vi "Sort SRs per Week(SubVI).vi"(8 "error in (no error)":errorcluster, 10 "Weeks":u8[](array[numeric]), 11 "Data Value Reference in":refnum<data-value>) -> (0 "error out":errorcluster, 3 "DVR Weekly/Country Data":refnum<data-value>)   [LabVIEW 2017, in "DS_Lib.lvlib" / "SRReportParser.lvlib"]
uses:
  Modules/Private Controls/Report Data Cluster.ctl
  Modules/Private Controls/Data Raw.ctl
  TypeDefs/WeeklyData.ctl
  SRReportParser.lvlib
  Modules/Data Operations.lvlib
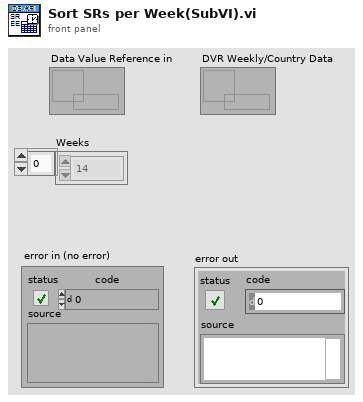
[diagram p1: front panel]
types:
  T1 = typedef "DS_Lib.lvlib/SRReportParser.lvlib/WeeklyData.ctl" = cluster{"Week":u8, "AE-Romania":T2[], "AE-Poland":T2[], "AE-Hungary":T2[], "AE-Czech and Slovakia":T2[]}
  T2 = typedef "Data Operations.lvlib/Data Raw.ctl" = cluster{"SR Number":string, "Status":string, "Summary":string, "AE Owner":string, "AE Group":string, "Contact":string, "SurveyData":cluster{"Resolution Time":dbl, "Total Satisfaction":dbl, "Response Time":dbl, "Courtesy":dbl, "Problem Solved":dbl, "Level of effort":dbl}, "Time Data":cluster{"Last Update Date":timestamp, "Creation Date":timestamp, "Creation week":u8, "Last Update Week":u8}}
  T3 = typedef "Data Operations.lvlib/Report Data Cluster.ctl" = cluster{"Headers":cluster{"Start Date":timestamp, "End Date":timestamp, "SR Status String":string[], "AE Owner String":string[]}, "Data":T2[]}
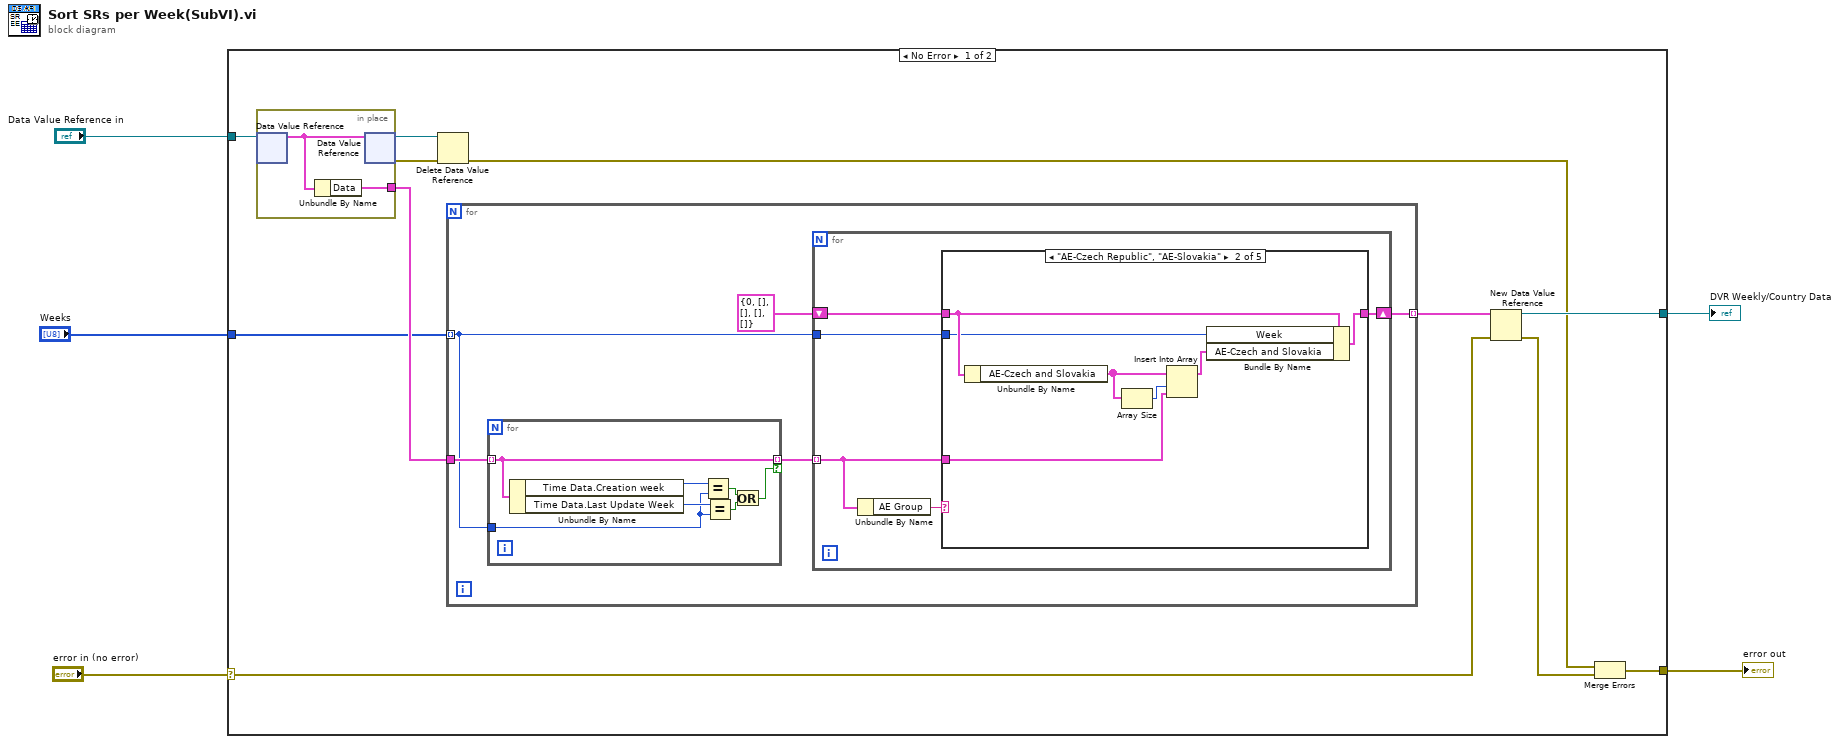
[diagram p0: block diagram]
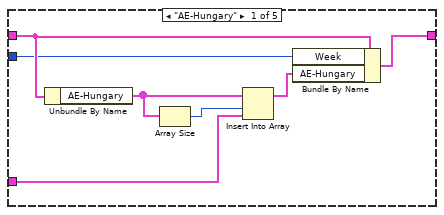
[diagram p2: hidden frame]
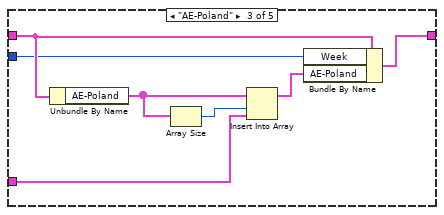
[diagram p3: hidden frame]
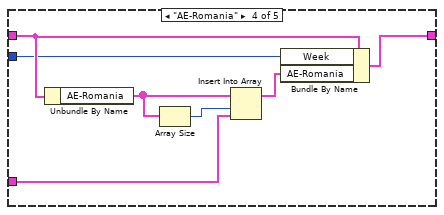
[diagram p4: hidden frame]
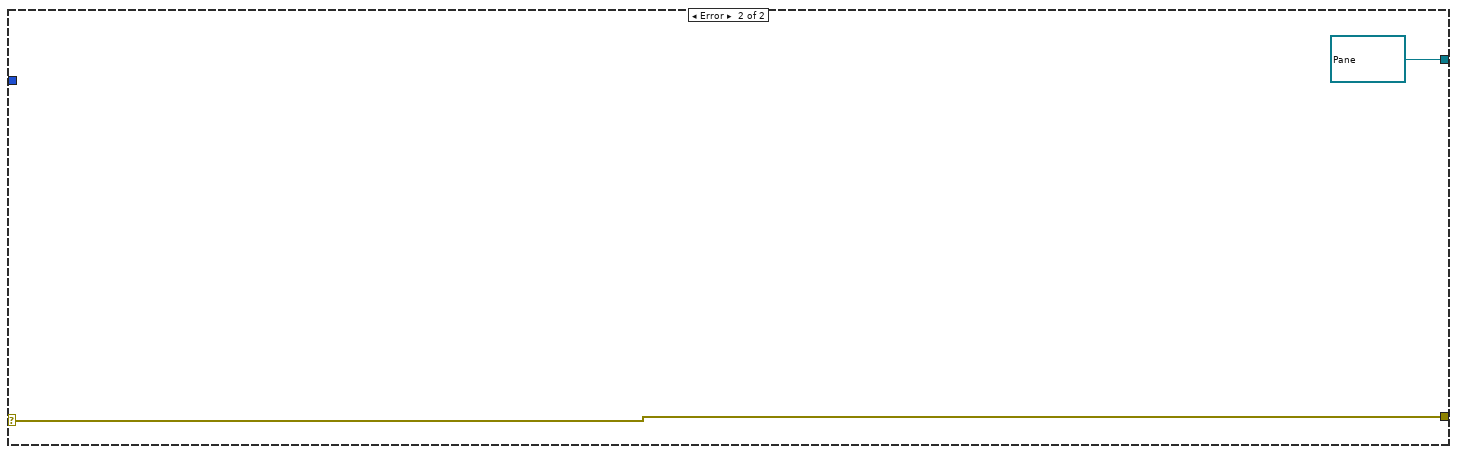
[diagram p6: hidden frame]
diagram:
  n1 = case shown="No Error" "error in (no error)" {
    selector: "error in (no error)" -> [w12 w66]
    tunnel: "Data Value Reference in" -> [w16 _]
    tunnel: [w15 w66] -> w4
    tunnel: "Weeks" -> [w13 _]
    tunnel: [w9 refnum<data-value> refnum ("data value reference")] -> w1
    frame No Error {
      n2 = in-place {
        in-place-border: [w63] -> w14
        n3 = in-place-dvr #1(w16) -> (w64:T3)  [unwired: 1 out]
        n4 = Unbundle By Name(w64) -> ("Data"=w63:T2[])
        n5 = in-place-dvr #1(w64) -> (w7:refnum<data-value>, w8:errorcluster)
      }
      n6 = Delete Data Value Reference(data value reference=w7, error in=w8) -> (error out=w6:errorcluster)  [unwired: 1 out]
      n7 = for {
        tunnel: w14 -> [w21]
        tunnel: w13 -> [w18] mode=indexing
        tunnel: [w17] -> w10 mode=indexing
        n8 = for {
          tunnel: w18 -> [w59]
          tunnel: w21 -> [w62] mode=indexing
          tunnel: [w62] -> w19 mode=indexing if=w56
          n9 = Unbundle By Name(w62) -> ("Time Data.Creation week"=w60:u8, "Time Data.Last Update Week"=w61:u8)
          n10 = Equal?(x=w60, y=w59) -> (x = y?=w58:bool)
          n11 = Equal?(x=w61, y=w59) -> (x = y?=w57:bool)
          n12 = Or(x=w58, y=w57) -> (x .or. y?=w56:bool)
        }
        n13 = for {
          shift-right: [w23] -> w17
          shift-left: T1 {"Week"=0, "AE-Romania"=[], "AE-Poland"=[], "AE-Hungary"=[], "AE-Czech and Slovakia"=[]} -> [w26]
          tunnel: w19 -> [w24] mode=indexing
          tunnel: w18 -> [w25]
          n14 = Unbundle By Name(w24) -> ("AE Group"=w22:string)
          n15 = case shown="\"AE-Czech Republic\", \"AE-Slovakia\"" w22 {
            tunnel: w26 -> [w30 w37 w44 w51 w55]
            tunnel: w25 -> [w28 w35 w42 w49 _]
            tunnel: w24 -> [w31 w38 w45 w52 _]
            tunnel: [w27 w34 w41 w48 w55] -> w23
            frame "AE-Hungary" {
              n16 = Unbundle By Name(w30) -> ("AE-Hungary"=w33:T2[])
              n17 = Array Size(array=w33) -> (size(s)=w32:i32)
              n18 = Insert Into Array(array=w33, index=w32, new element=w31) -> (w29:T2[])
              n19 = Bundle By Name(cluster=w30, "Week"=w28, "AE-Hungary"=w29) -> (w27:T1)
            }
            frame "AE-Czech Republic", "AE-Slovakia" {
              n20 = Unbundle By Name(w37) -> ("AE-Czech and Slovakia"=w40:T2[])
              n21 = Array Size(array=w40) -> (size(s)=w39:i32)
              n22 = Insert Into Array(array=w40, index=w39, new element=w38) -> (w36:T2[])
              n23 = Bundle By Name(cluster=w37, "Week"=w35, "AE-Czech and Slovakia"=w36) -> (w34:T1)
            }
            frame "AE-Poland" {
              n24 = Unbundle By Name(w44) -> ("AE-Poland"=w47:T2[])
              n25 = Array Size(array=w47) -> (size(s)=w46:i32)
              n26 = Insert Into Array(array=w47, index=w46, new element=w45) -> (w43:T2[])
              n27 = Bundle By Name(cluster=w44, "Week"=w42, "AE-Poland"=w43) -> (w41:T1)
            }
            frame "AE-Romania" {
              n28 = Unbundle By Name(w51) -> ("AE-Romania"=w54:T2[])
              n29 = Array Size(array=w54) -> (size(s)=w53:i32)
              n30 = Insert Into Array(array=w54, index=w53, new element=w52) -> (w50:T2[])
              n31 = Bundle By Name(cluster=w51, "Week"=w49, "AE-Romania"=w50) -> (w48:T1)
            }
            frame "Default Case", Default {
            }
          }
        }
      }
      n32 = New Data Value Reference(data value=w10, error in=w12) -> (data value reference=w9:refnum<data-value>, error out=w11:errorcluster)
      n33 = Merge Errors(w6, w11) -> (w15:errorcluster)
    }
    frame Error {
    }
  }
  "error out" <- w4
  "DVR Weekly/Country Data" <- w1
